vi "GetPilotLocs (SubVI).vi"(0 "sym #":i16, 1 "pilot_offset_freq":i16, 2 "pilot_offset_time":i16, 3 "sc_pilot":i16, 4 "pilot_start":i16) -> (5 "Array":i32[](array[numeric]))   [LabVIEW 2015]
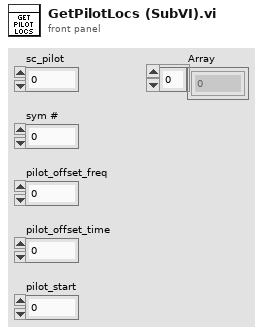
[diagram p1: front panel]
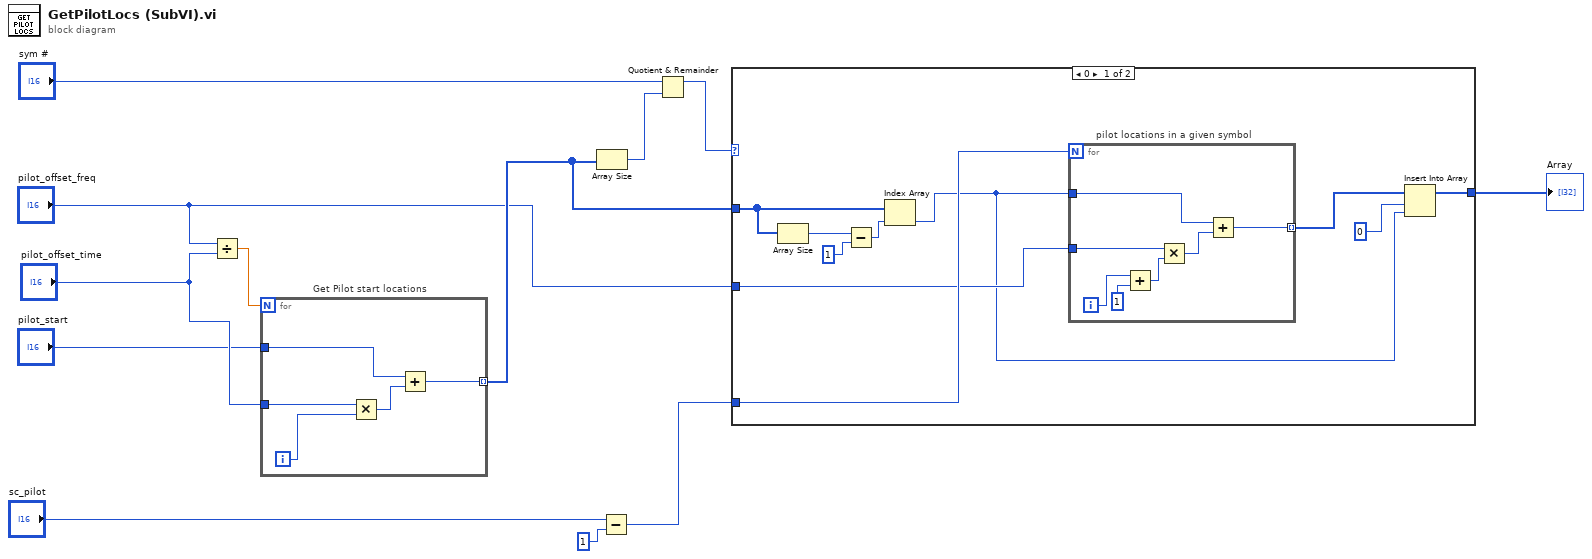
[diagram p0: block diagram]
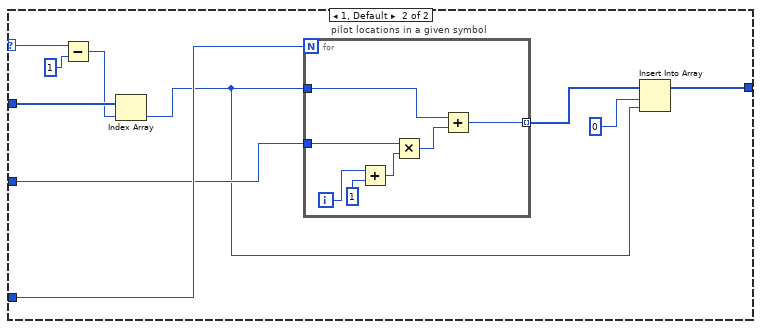
[diagram p2: hidden frame]
diagram:
  n1 = Divide(x="pilot_offset_freq", y="pilot_offset_time") -> (x/y=w10:dbl)
  n2 = for "Get Pilot start locations" {
    N: w10 -> [_]
    tunnel: [w16] -> w12 mode=indexing
    tunnel: "pilot_start" -> [w15]
    tunnel: "pilot_offset_time" -> [w13]
    i -> [w14]
    n3 = Multiply(x=w13, y=w14) -> (x*y=w17:i32)
    n4 = Add(x=w15, y=w17) -> (x+y=w16:i32)
  }
  n5 = Array Size(array=w12) -> (size(s)=w2:i32)
  n6 = Subtract(x="sc_pilot", y=i16 1) -> (x-y=w5:i16)
  n7 = Quotient & Remainder(x="sym #", y=w2) -> (x-y*floor(x/y)=w6:i32)  [unwired: 1 out]
  n8 = case shown="0" w6 {
    selector: w6 -> [_ w36]
    tunnel: w5 -> [w27 w41]
    tunnel: "pilot_offset_freq" -> [w26 w40]
    tunnel: [w23 w42] -> w7
    tunnel: w12 -> [w20 w38]
    frame 0 {
      n9 = Array Size(array=w20) -> (size(s)=w19:i32)
      n10 = Subtract(x=w19, y=1) -> (x-y=w21:i32)
      n11 = Index Array(array=w20, index=w21) -> (element=w18:i32)
      n12 = for "pilot locations in a given symbol" {
        N: w27 -> [_]
        tunnel: w26 -> [w30]
        tunnel: [w29] -> w24 mode=indexing
        tunnel: w18 -> [w28]
        i -> [w33]
        n13 = Add(x=w33, y=1) -> (x+y=w31:i32)
        n14 = Multiply(x=w30, y=w31) -> (x*y=w34:i32)
        n15 = Add(x=w28, y=w34) -> (x+y=w29:i32)
      }
      n16 = Insert Into Array(array=w24, index=0, new element=w18) -> (w23:i32[])
    }
    frame 1, Default {
      n17 = Subtract(x=w36, y=i16 1) -> (x-y=w35:i32)
      n18 = Index Array(array=w38, index=w35) -> (element=w39:i32)
      n19 = for "pilot locations in a given symbol" {
        N: w41 -> [_]
        tunnel: w40 -> [w47]
        tunnel: [w46] -> w44 mode=indexing
        tunnel: w39 -> [w45]
        i -> [w50]
        n20 = Add(x=w50, y=1) -> (x+y=w48:i32)
        n21 = Multiply(x=w47, y=w48) -> (x*y=w51:i32)
        n22 = Add(x=w45, y=w51) -> (x+y=w46:i32)
      }
      n23 = Insert Into Array(array=w44, index=0, new element=w39) -> (w42:i32[])
    }
  }
  "Array" <- w7
